vi "Periodic Tasks.vi"(8 "error in":errorcluster) -> ()   [LabVIEW 2019]
doc: "This VI runs in parallel to other tasks. It can contain as many user-defined periodic loops as you need. These can carry out PID or other sorts of timed response."
uses:
  Robot Global Data.vi
  <vilib>/addons/control/pid/NI_PID_pid.lvlib
  <vilib>/Rock Robotics/Network Tables/NT Write Number.vi
  <vilib>/Rock Robotics/Network Tables/NT Read Number.vi
  <vilib>/addons/control/pid/pid.llb/PID (DBL).vi
  <vilib>/Rock Robotics/WPI/RobotDrive/WPI_RobotDriveArcadeDrive_Standard(NoSaturation).vi
  <vilib>/Rock Robotics/Network Tables/NT Write Boolean.vi
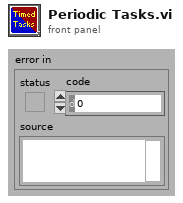
[diagram p1: front panel]
types:
  T1 = typedef "WPI_JoystickDevRef.ctl" = cluster{"Device":T2}
  T2 = typedef "WPI_JoystickDeviceEnum.ctl" = enum16{"USB 0", "USB 1", "USB 2", "USB 3", "USB 4", "USB 5"}
  T3 = typedef "WPI_RobotDriveDevRef.ctl" = cluster{"DevStatus":errorcluster, "Motors[]":T4[], "Square Inputs":bool, "Max Output":dbl}
  T4 = typedef "WPI_MotorControlDeviceRef.ctl" = cluster{"DeviceStatus":errorcluster, "Type":T5, "PWM":cluster{"PWM Channel":T6, "DeadBand":T7}, "CAN":cluster{"Device Number":u8, "SetOutput VI Ref":variant, "GetOutput VI Ref":variant, "Enable VI Ref":variant, "Disable VI Ref":variant, "Data":variant}, "Invert":bool, "DIO PWM":cluster{"PWM \"Enable\" Channel":T6, "DIOChannel":T8, "PWM Rate":dbl}}
  T5 = typedef "WPI_MotorControlType.ctl" = enum16{"PWM", "CAN", "DIO PWM"}
  T6 = typedef "FPGA_DIOPWMChannel.ctl" = enum8{"PWM 0", "PWM 1", "PWM 2", "PWM 3", "PWM 4", "PWM 5", "PWM 6", "PWM 7", "PWM 8", "PWM 9", "PWM MXP 0", "PWM MXP 1", "PWM MXP 2", "PWM MXP 3", "PWM MXP 4", "PWM MXP 5", "PWM MXP 6", "PWM MXP 7", "PWM MXP 8", "PWM MXP 9", "Invalid"}
  T7 = typedef "WPI_PWMDeadband.ctl" = cluster{"Name":string, "maxPositivePwm":i32, "minPositivePwm":i32, "centerPwm":i32, "maxNegativePwm":i32, "minNegativePwm":i32, "angularRange":u16}
  T8 = typedef "FPGA_DIOChannel.ctl" = enum8{"DIO 0", "DIO 1", "DIO 2", "DIO 3", "DIO 4", "DIO 5", "DIO 6", "DIO 7", "DIO 8", "DIO 9", "DIO MXP 0", "DIO MXP 1", "DIO MXP 2", "DIO MXP 3", "DIO MXP 4", "DIO MXP 5", "DIO MXP 6", "DIO MXP 7", "DIO MXP 8", "DIO MXP 9", "DIO MXP 10", "DIO MXP 11", "DIO MXP 12", "DIO MXP 13", "DIO MXP 14", "DIO MXP 15", "SPI Port CS1", "SPI Port CS2", "SPI Port CS3", "SPI Port MISO", "SPI Port MOSI", "Invalid"}
  T9 = cluster{"JoystickDevRef":T1, "RobotDriveDevRef":T3}
  T10 = cluster{"proportional gain":dbl, "integral time":dbl, "derivative time":dbl}
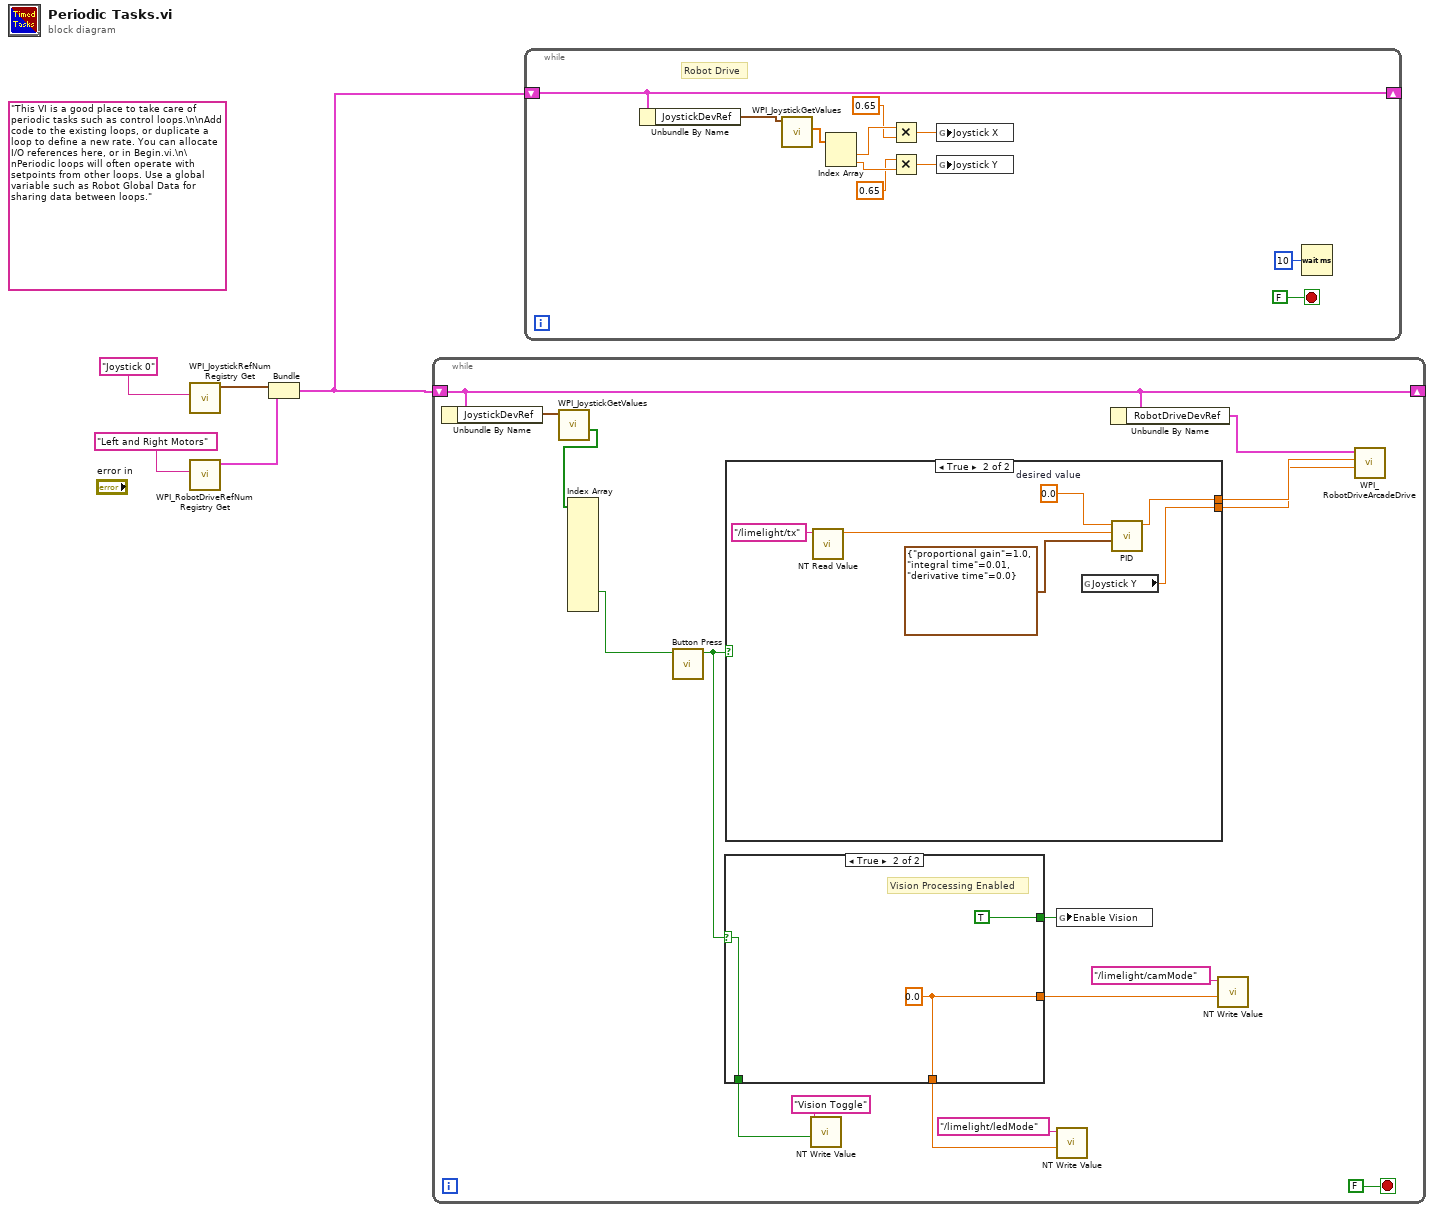
[diagram p0: block diagram]
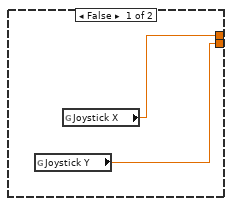
[diagram p2: hidden frame]
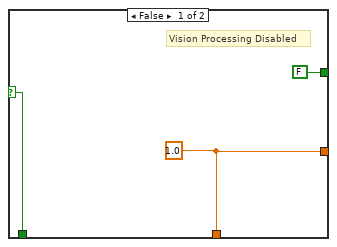
[diagram p3: hidden frame]
diagram:
  (unwired) "This VI is a good place to take care of periodic tasks such as control loops.\n\nAdd code to the existing loops, or duplicate a loop to define a new rate. You can allocate I/O references here, or in Begin.vi.\n\nPeriodic loops will often operate with setpoints from other loops. Use a global variable such as Robot Global Data for sharing data between loops."
  n1 = call <vilib>:"WPI_JoystickRefNum Registry Get.vi"("refnum name"="Joystick 0") -> ("JoystickDevRef"=w3:T1)  [unwired: 1 in, 9 out]
  n2 = call <vilib>:"WPI_RobotDriveRefNum Registry Get.vi"("refnum name"="Left and Right Motors") -> ("RobotDriveDevRef"=w2:T3)  [unwired: 1 in, 9 out]
  n3 = Bundle("JoystickDevRef"=w3, "RobotDriveDevRef"=w2) -> (w1:T9)  [unwired: 1 out]
  n4 = while {
    shift-right: [w16] -> _
    shift-left: w1 -> [w16]
    stop <- FALSE stop-if-true
    n5 = Unbundle By Name(w16) -> ("JoystickDevRef"=w15:T1)
    n6 = call <vilib>:"WPI_JoystickGetValues.vi"("JoystickDevRef"=w15) -> ("Buttons"=w14:bool[])  [unwired: 6 in, 4 out]
    n7 = Index Array(array=w14) -> (element #10=w7:bool)  [unwired: 12 in, 11 out]
    n8 = call "Button Press.vi"("Button"=w7) -> ("Button Pressed?"=w6:bool)  [unwired: 10 in]
    n9 = case shown="True" w6 {
      selector: w6 -> [w30 w33]
      tunnel: [FALSE ("Enable Vision") TRUE ("Enable Vision")] -> w20
      tunnel: [w31 w34] -> w12
      tunnel: [w31 w34] -> w10
      tunnel: [w30 w33] -> w8
      frame False {
        w31 = 1.0 ("Numeric")
        # "Vision Processing Disabled"
      }
      frame True {
        w34 = 0.0 ("Numeric")
        # "Vision Processing Enabled"
      }
    }
    n10 = case shown="True" w6 {
      tunnel: [w23 w27] -> w18
      tunnel: [w22 w24] -> w17
      frame False {
        n11 = global read "Robot Global Data.vi" "Joystick Y"() -> (w22:dbl)
        n12 = global read "Robot Global Data.vi" "Joystick X"() -> (w23:dbl)
      }
      frame True {
        w25 = 0.0  # desired value
        n13 = call-poly <vilib>:"NT Read Value.vi"("Name"="/limelight/tx") -> ("Numeric"=w28:dbl)  [unwired: 9 in, 1 out]
        n14 = global read "Robot Global Data.vi" "Joystick Y"() -> (w24:dbl)
        n15 = call-poly <vilib>:"PID.vi"("PID gains"=T10 {"proportional gain"=1.0, "integral time"=0.01, "derivative time"=0.0}, "process variable"=w28, "setpoint"=w25) -> ("output"=w27:dbl)  [unwired: 7 in, 1 out]
      }
    }
    n16 = call-poly <vilib>:"NT Write Value.vi"("Boolean"=w8, "Name"="Vision Toggle") -> ()  [unwired: 9 in, 1 out]
    n17 = global write "Robot Global Data.vi" "Enable Vision"(w20) -> ()
    n18 = call-poly <vilib>:"NT Write Value.vi"("Numeric"=w10, "Name"="/limelight/ledMode") -> ()  [unwired: 9 in, 1 out]
    n19 = Unbundle By Name(w16) -> ("RobotDriveDevRef"=w19:T3)
    n20 = call-poly <vilib>:"NT Write Value.vi"("Numeric"=w12, "Name"="/limelight/camMode") -> ()  [unwired: 9 in, 1 out]
    n21 = call-poly <vilib>:"WPI_RobotDriveArcadeDrive.vi"("Y axis value"=w17, "X axis value"=w18, "RobotDriveDevRef"=w19) -> ()  [unwired: 6 in, 3 out]
  }
  n22 = while {
    shift-right: [w45] -> _
    shift-left: w1 -> [w45]
    stop <- FALSE stop-if-true
    # "Robot Drive"
    n23 = Unbundle By Name(w45) -> ("JoystickDevRef"=w43:T1)
    n24 = call <vilib>:"WPI_JoystickGetValues.vi"("JoystickDevRef"=w43) -> ("Axes"=w42:dbl[])  [unwired: 6 in, 4 out]
    n25 = Index Array(array=w42) -> (element #1=w41:dbl, element #2=w39:dbl)  [unwired: 2 in]
    n26 = Multiply(x=w41, y=0.65) -> (x*y=w37:dbl)
    n27 = Multiply(x=0.65, y=w39) -> (x*y=w36:dbl)
    n28 = global write "Robot Global Data.vi" "Joystick X"(w37) -> ()
    n29 = global write "Robot Global Data.vi" "Joystick Y"(w36) -> ()
    n30 = Wait (ms)(milliseconds to wait=u32 10) -> ()  [unwired: 1 out]
  }
